vi "Pass or Fail.vi"(6 "Numeric in":i32, 7 "Ligne à modifier":string[][](array[string]), 8 "error in (no error)":errorcluster, 9 "Nom test":string, 10 "String":string, 11 "Boolean":bool) -> (0 "error out":errorcluster, 2 "Numeric out":i32, 3 "tableau sortie":string)   [LabVIEW 2017]
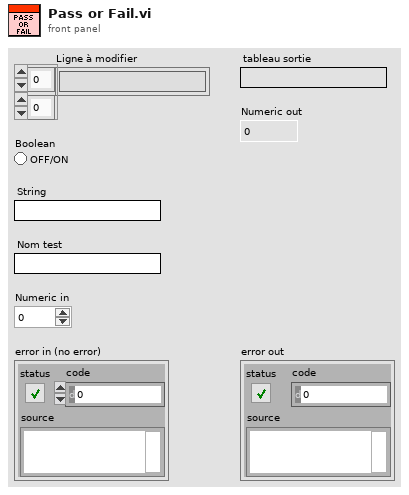
[diagram p1: front panel]
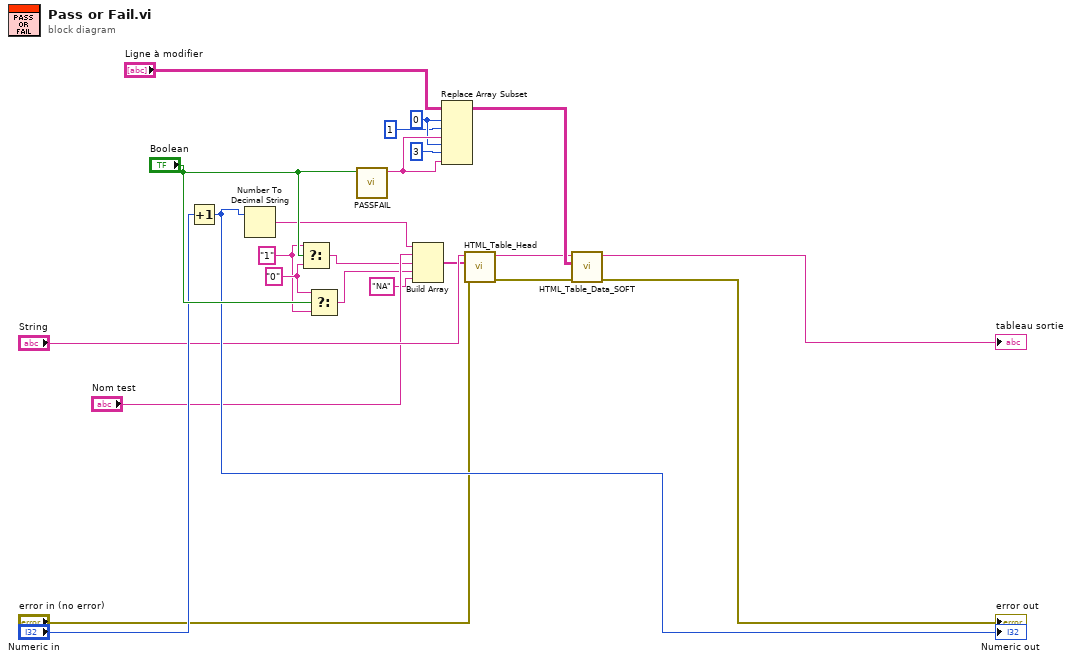
[diagram p0: block diagram]
diagram:
  w22 = 0 ("indice désactivé (ligne)")
  w5 = "0" ("cas faux")
  w4 = "1"
  n1 = Increment(x="Numeric in") -> (x+1=w16:i32)
  "Numeric out" <- w16
  n2 = Number To Decimal String(number=w16) -> (decimal integer string=w9:string)  [unwired: 1 in]
  n3 = Select(t=w4, s="Boolean", f=w5) -> (s? t:f=w6:string)
  n4 = Select(t=w5, s="Boolean", f=w4) -> (s? t:f=w3:string)
  n5 = call "PASSFAIL.vi"("E"="Boolean") -> ("S"=w23:string)  [unwired: 10 in]
  n6 = Build Array(w9, "Nom test", w6, w3, "NA" ("élément")) -> (w2:string[])
  n7 = Replace Array Subset(array="Ligne à modifier", new element #1=w23, index (row) #1=w22, index (col) #1=1 ("indice désactivé (col)"), new element #2=w23, index (row) #2=w22, index (col) #2=3 ("disabled index (col)")) -> (w18:string[][])
  n8 = call "HTML_Table_Head.vi"("entrée d'erreur (pas d'erreur)"="error in (no error)", "Tableau"=w2, "chaîne en entrée"="String") -> ("sortie d'erreur"=w7:errorcluster, "result string"=w8:string)  [unwired: 7 in]
  n9 = call "HTML_Table_Data_SOFT.vi"("entrée d'erreur (pas d'erreur)"=w7, "Tableau"=w18, "chaîne en entrée"=w8) -> ("sortie d'erreur"=→"error out":errorcluster, "result string"=→"tableau sortie":string)  [unwired: 7 in]
